vi "Arcazde.vi"(2 "y":dbl, 3 "Boolean":bool, 4 "x":dbl) -> (0 "RightSide":dbl, 1 "LeftSide":dbl)   [LabVIEW 2012]
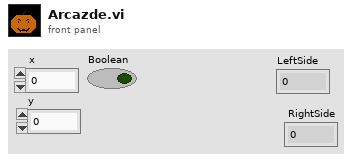
[diagram p1: front panel]
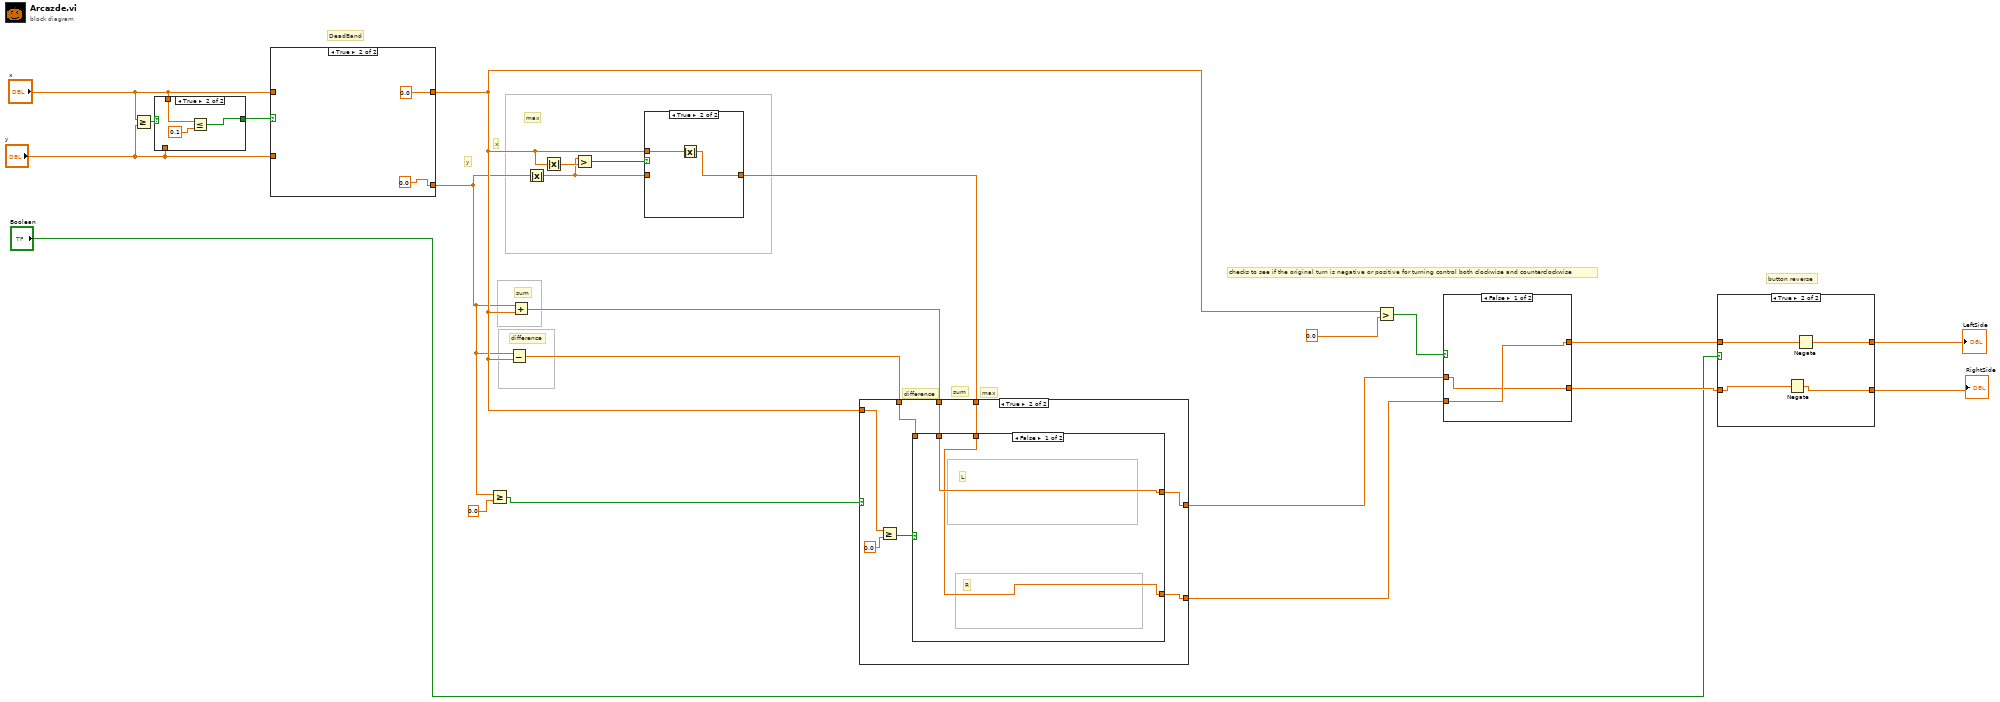
[diagram p0: block diagram]
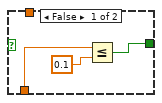
[diagram p2: hidden frame]
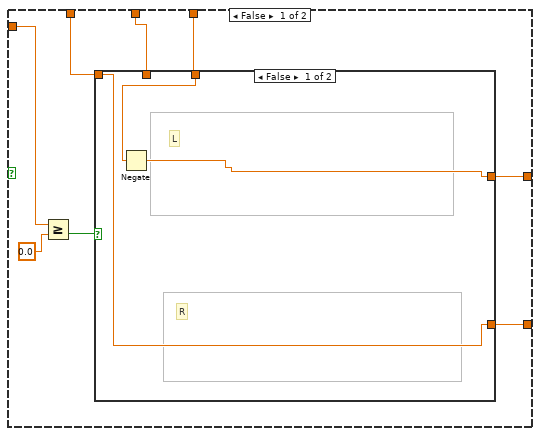
[diagram p6: hidden frame]
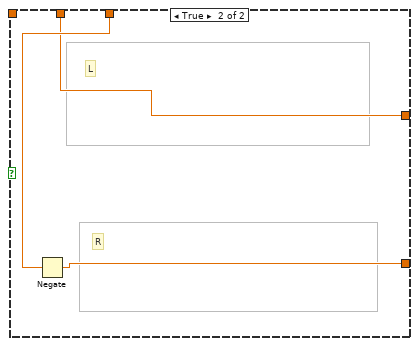
[diagram p7: hidden frame]
diagram:
  # "DeadBand"
  # "button reverse"
  # "checks to see if the original turn is negative or positive for turning control both clockwise and counterclockwise"
  # "difference"
  # "sum"
  # "max"
  # "difference"
  # "sum"
  # "x"
  # "y"
  # "max"
  n1 = Greater Or Equal?(x="x", y="y") -> (x >= y?=w4:bool)
  n2 = case shown="True" w4 {
    tunnel: "x" -> [_ w29]
    tunnel: "y" -> [w25 _]
    tunnel: [w24 w27] -> w1
    frame False {
      n3 = Less Or Equal?(x=w25, y=0.1) -> (x <= y?=w24:bool)
    }
    frame True {
      n4 = Less Or Equal?(x=w29, y=0.1) -> (x <= y?=w27:bool)
    }
  }
  n5 = case shown="True" w1 {
    tunnel: [w31 0.0 ("x")] -> w6
    tunnel: "x" -> [w31 _]
    tunnel: [w30 0.0 ("x")] -> w5
    tunnel: "y" -> [w30 _]
    frame False {
    }
    frame True {
    }
  }
  n6 = Greater Or Equal?(x=w5, y=0.0) -> (x >= y?=w19:bool)
  n7 = Subtract(x=w5, y=w6) -> (x-y=w17:dbl)
  n8 = Add(x=w5, y=w6) -> (x+y=w16:dbl)
  n9 = Absolute Value(x=w5) -> (abs(x)=w22:dbl)
  n10 = Absolute Value(x=w6) -> (abs(x)=w23:dbl)
  n11 = Greater?(x=w22, y=w23) -> (0:w21:bool)
  n12 = case shown="True" w21 {
    tunnel: w22 -> [w34 _]
    tunnel: [w34 w35] -> w18
    tunnel: w6 -> [_ w36]
    frame False {
    }
    frame True {
      n13 = Absolute Value(x=w36) -> (abs(x)=w35:dbl)
    }
  }
  n14 = case shown="True" w19 {
    tunnel: w6 -> [w42 w57]
    tunnel: w18 -> [w41 w55]
    tunnel: w17 -> [w40 w54]
    tunnel: w16 -> [w39 w53]
    tunnel: [w38 w52] -> w13
    tunnel: [w37 w51] -> w12
    frame False {
      n15 = Greater Or Equal?(x=w42, y=0.0) -> (x >= y?=w44:bool)
      n16 = case shown="False" w44 {
        tunnel: w41 -> [w47 w50]
        tunnel: w40 -> [w45 _]
        tunnel: w39 -> [_ w49]
        tunnel: [w46 w49] -> w38
        tunnel: [w45 w48] -> w37
        frame False {
          # "L"
          # "R"
          n17 = Negate(x=w47) -> (-x=w46:dbl)
        }
        frame True {
          # "L"
          # "R"
          n18 = Negate(x=w50) -> (-x=w48:dbl)
        }
      }
    }
    frame True {
      n19 = Greater Or Equal?(x=w57, y=0.0) -> (x >= y?=w58:bool)
      n20 = case shown="False" w58 {
        tunnel: w55 -> [w59 w62]
        tunnel: w54 -> [_ w61]
        tunnel: w53 -> [w60 _]
        tunnel: [w60 w62] -> w52
        tunnel: [w59 w61] -> w51
        frame False {
          # "L"
          # "R"
        }
        frame True {
          # "L"
          # "R"
        }
      }
    }
  }
  n21 = Greater?(x=w6, y=0.0) -> (0:w15:bool)
  n22 = case shown="False" w15 {
    tunnel: [w63 w66] -> w10
    tunnel: [w64 w65] -> w11
    tunnel: w13 -> [w63 w65]
    tunnel: w12 -> [w64 w66]
    frame False {
    }
    frame True {
    }
  }
  n23 = case shown="True" "Boolean" {
    tunnel: w11 -> [w68 w72]
    tunnel: w10 -> [w67 w69]
    tunnel: [w68 w71] -> w9
    tunnel: [w67 w70] -> w8
    frame False {
    }
    frame True {
      n24 = Negate(x=w69) -> (-x=w70:dbl)
      n25 = Negate(x=w72) -> (-x=w71:dbl)
    }
  }
  "LeftSide" <- w9
  "RightSide" <- w8
